vi "FTW-File-FileVersion.vi"(0 "Filepath":path, 11 "error in":errorcluster) -> (4 "File Version":string, 6 "Product Version":string, 8 "File Description":string, 10 "Legal Copyright":string, 15 "error out":errorcluster)   [LabVIEW 2014]
panel:
  # "Inputs"
  # "Outputs"
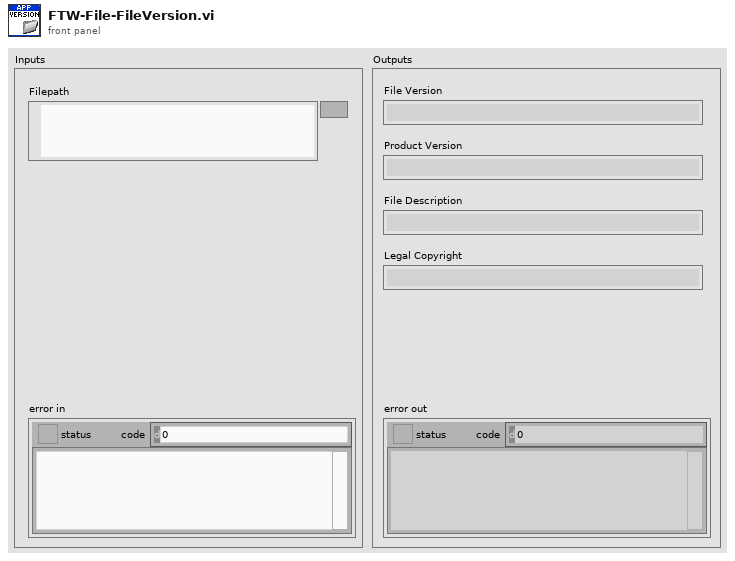
[diagram p1: front panel]
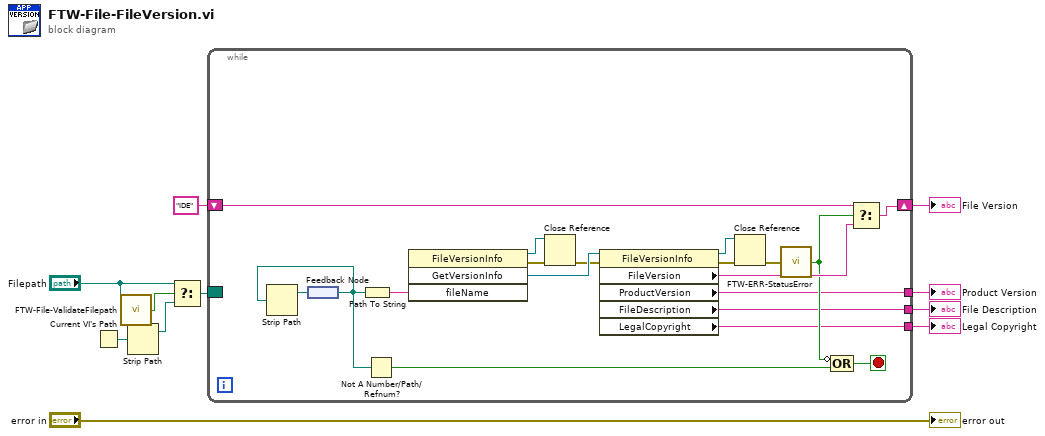
[diagram p0: block diagram]
diagram:
  n1 = Current VI's Path() -> (path=w6:path)
  n2 = call "FTW-File-ValidateFilepath.vi"("Filepath"="Filepath") -> ("Valid?"=w8:bool)
  n3 = Strip Path(path=w6) -> (stripped path=w5:path)  [unwired: 1 out]
  n4 = Select(t="Filepath", s=w8, f=w5) -> (s? t:f=w7:path)
  n5 = while {
    border: w7 -> [_]
    shift-right: [w27] -> w9
    shift-left: "IDE" ("File Version Info") -> [w28]
    tunnel: [w15] -> w3
    tunnel: [w13] -> w2
    tunnel: [w12] -> w1
    stop <- w29 stop-if-true
    n6 = feedback #1() -> (w14:path)
    n7 = Strip Path(path=w14) -> (stripped path=w23:path)  [unwired: 1 out]
    n8 = feedback-in #1(w23) -> ()
    n9 = Path To String(path=w14) -> (string=w26:string)
    n10 = Not A Number/Path/Refnum?(number/path/refnum=w14) -> (NaN/Path/Refnum?=w30:bool)
    n11 = invoke class="FileVersionInfo" method="GetVersionInfo"("fileName"=w26) -> (reference out=w18:refnum<k24>, error out=w17:errorcluster, "GetVersionInfo"=w22:refnum<k24>)  [unwired: 3 in, 1 out]
    n12 = Close Reference(reference=w18, error in (no error)=w17) -> (error out=w16:errorcluster)
    n13 = property class="FileVersionInfo"(reference=w22, error in=w16) -> (reference out=w21:refnum<k24>, error out=w20:errorcluster, "FileVersion"=w25:string, "ProductVersion"=w15:string, "FileDescription"=w13:string, "LegalCopyright"=w12:string)
    n14 = Close Reference(reference=w21, error in (no error)=w20) -> (error out=w19:errorcluster)
    n15 = call "FTW-ERR-StatusError.vi"("error to check"=w19) -> ("Error?"=w24:bool)
    n16 = Compound Arithmetic op=OR(invert w24, w30) -> (w29:bool)
    n17 = Select(t=w28, s=w24, f=w25) -> (s? t:f=w27:string)
  }
  "File Version" <- w9
  "Product Version" <- w3
  "File Description" <- w2
  "Legal Copyright" <- w1
  "error out" <- "error in"
